vi "8Queen_quest2.vi"() -> ()   [LabVIEW 2012]
panel:
  out "Attempts":i32
  out "sec_past":dbl format="%#_4g"
  out "Solutions":i32
  in  "stop":bool
  in  "soln_dsp":i32=1
  out "board":bool[][](array[boolean])
  out "all_soln_out":i32[][](array[numeric])
  in  "Q_num":i32=9
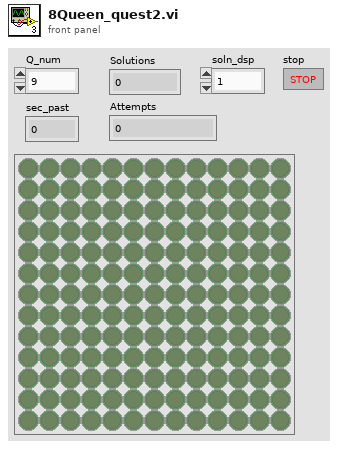
[diagram p1: front panel]
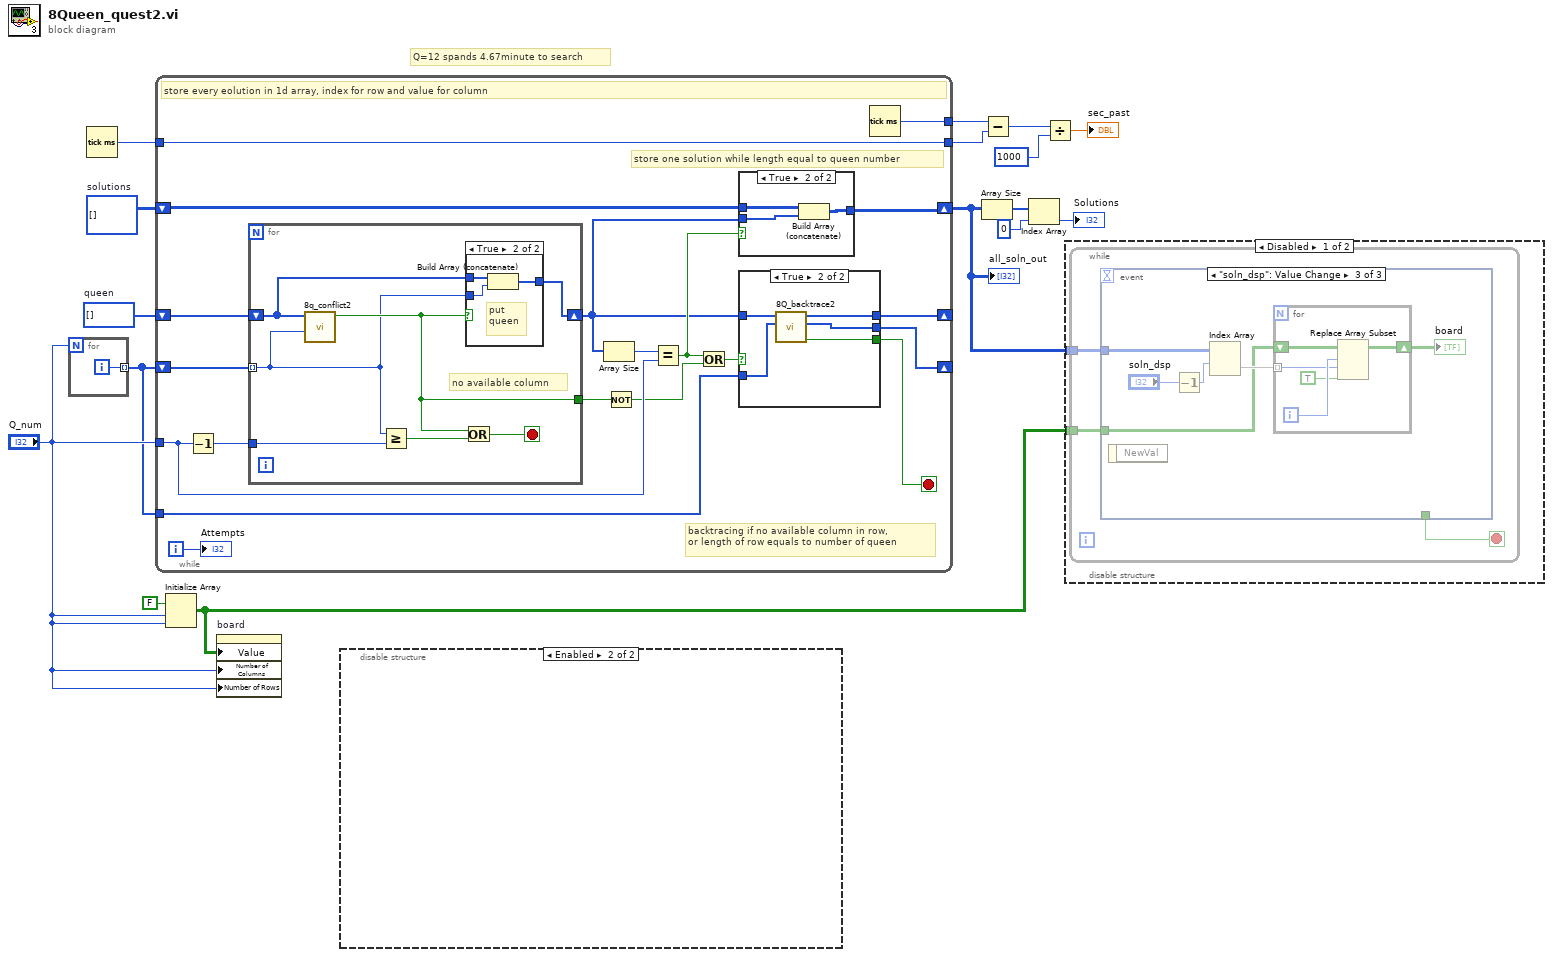
[diagram p0: block diagram]
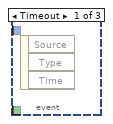
[diagram p2: hidden frame]
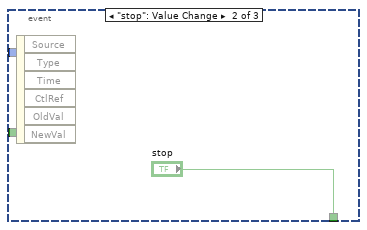
[diagram p3: hidden frame]
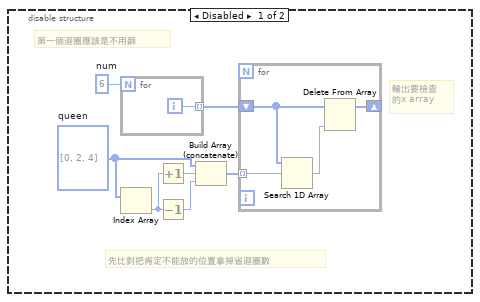
[diagram p5: hidden frame]
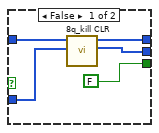
[diagram p8: hidden frame]
diagram:
  w15 = i32[] []  # queen
  w16 = i32[][] []  # solutions
  # "Q=12 spands 4.67minute to search"
  n1 = for {
    N: "Q_num" -> [_]
    tunnel: [w17] -> w1 mode=indexing
    i -> [w17]
  }
  n2 = Tick Count (ms)() -> (millisecond timer value=w4:u32)
  n3 = while {
    shift-right: [w33] -> _
    shift-left: w15 -> [w26]
    shift-right: [w27] -> _
    shift-left: w1 -> [w25]
    tunnel: "Q_num" -> [w31]
    shift-right: [w18] -> w14
    shift-left: w16 -> [w19]
    tunnel: [w30] -> w5
    tunnel: w4 -> [w29]
    tunnel: [w29] -> w3
    tunnel: w1 -> [w28]
    i -> [w22]
    stop <- w34 stop-if-true
    # "store one solution while length equal to queen number"
    # "backtracing if no available column in row,\nor length of row equals to number of queen"
    # "store every eolution in 1d array, index for row and value for column"
    n4 = Decrement(x=w31) -> (x-1=w32:i32)
    n5 = for {
      shift-right: [w41] -> w20
      shift-left: w26 -> [w42]
      tunnel: w32 -> [w47]
      tunnel: [w44] -> w23
      tunnel: w25 -> [w43] mode=indexing
      stop <- w45 stop-if-true
      # "no available column"
      n6 = call "8q_conflict2.vi"("nextX"=w43, "State"=w42) -> ("Available"=w44:bool)  [unwired: 9 in]
      n7 = Greater Or Equal?(x=w43, y=w47) -> (x >= y?=w46:bool)
      n8 = Or(x=w44, y=w46) -> (x .or. y?=w45:bool)
      n9 = case shown="True" w44 {
        tunnel: w43 -> [_ w51]
        tunnel: w42 -> [w48 w50]
        tunnel: [w48 w49] -> w41
        frame False {
        }
        frame True {
          # "put\nqueen"
          n10 = Build Array (concatenate)(w50, w51) -> (w49:i32[])
        }
      }
    }
    n11 = Array Size(array=w20) -> (size(s)=w36:i32)
    n12 = Not(x=w23) -> (.not. x?=w24:bool)
    n13 = Equal?(x=w36, y=w31) -> (x = y?=w21:bool)
    n14 = Or(x=w21, y=w24) -> (x .or. y?=w35:bool)
    n15 = case shown="True" w21 {
      tunnel: w20 -> [_ w40]
      tunnel: w19 -> [w37 w39]
      tunnel: [w37 w38] -> w18
      frame False {
      }
      frame True {
        n16 = Build Array (concatenate)(w39, w40) -> (w38:i32[][])
      }
    }
    n17 = case "backtracing" shown="True" w35 {
      tunnel: [w52 w59] -> w27
      tunnel: w20 -> [w54 w61]
      tunnel: [w53 w60] -> w33
      tunnel: [FALSE ("<0_stop") w58] -> w34
      tunnel: w28 -> [w55 w57]
      frame False {
        n18 = call "8q_kill CLR.vi"("nextX in"=w55, "queen in"=w54) -> ("nextX"=w52:i32[], "queen"=w53:i32[])  [unwired: 8 in]
      }
      frame True {
        n19 = call "8Q_backtrace2.vi"("all_x"=w57, "BT_bfr"=w61) -> ("<0_stop"=w58:bool, "next_start"=w59:i32[], "BT_result"=w60:i32[])  [unwired: 7 in]
      }
    }
    n20 = Tick Count (ms)() -> (millisecond timer value=w30:u32)
    "Attempts" <- w22
  }
  "all_soln_out" <- w14
  n21 = Initialize Array(FALSE, "Q_num", "Q_num") -> (w9:bool[][])
  n22 = property on="board" class="Arr (strict)"("Value"=w9, "Number of Columns"="Q_num", "Number of Rows"="Q_num") -> ()  [unwired: 2 in, 2 out]
  n23 = disable-structure shown="Enabled" {
    frame Disabled {
      w68 = 6  # num
      w65 = i32[] [0, 2, 4]  # queen
      # "第一個迴圈應該是不用篩"
      # "輸出要檢查\n的x array"
      # "先比對把肯定不能放的位置拿掉省迴圈數"
      n24 = for {
        N: w68 -> [_]
        tunnel: [w73] -> w67 mode=indexing
        i -> [w73]
      }
      n25 = Index Array(array=w65) -> (element=w63:i32)  [unwired: 1 in]
      n26 = Increment(x=w63) -> (x+1=w66:i32)
      n27 = Decrement(x=w63) -> (x-1=w64:i32)
      n28 = Build Array (concatenate)(w65, w66, w64) -> (w62:i32[])
      n29 = for {
        tunnel: w62 -> [w72] mode=indexing
        shift-right: [w69] -> _
        shift-left: w67 -> [w70]
        n30 = Search 1D Array(1D array=w70, element=w72) -> (index of element=w71:i32)  [unwired: 1 in]
        n31 = Delete From Array(array=w70, index=w71) -> (array with subset deleted=w69:i32[])  [unwired: 1 in, 1 out]
      }
    }
    frame Enabled {
    }
  }
  n32 = Array Size(array=w14) -> (size(s)=w13:i32[])
  n33 = Subtract(x=w5, y=w3) -> (x-y=w8:u32)
  n34 = Index Array(array=w13, index=0) -> (element=→"Solutions":i32)
  n35 = Divide(x=w8, y=u32 1000) -> (x/y=→"sec_past":dbl)
  n36 = disable-structure shown="Disabled" {
    disable-tunnel: w14 -> [w75 _]
    disable-tunnel: w9 -> [w74 _]
    frame Disabled {
      n37 = while {
        tunnel: w75 -> [w78]
        tunnel: w74 -> [w76]
        stop <- w77 stop-if-true
        n38 = event shown="[2] \"soln_dsp\": Value Change" {
          selector: _ -> [_ _ _]
          dyn-events: _ -> [_ _ _]
          timeout: _ -> [_ _ _]
          tunnel: w78 -> [_ _ w85]
          tunnel: [_ "stop" _] -> w77
          tunnel: w76 -> [_ _ w80]
          event Timeout {
            n39 = event-data() -> ()  [unwired: 1 in, 3 out]
          }
          event "stop": Value Change {
            n40 = event-data() -> ()  [unwired: 1 in, 6 out]
          }
          event "soln_dsp": Value Change {
            n41 = event-data() -> ()  [unwired: 1 in, 1 out]
            n42 = Decrement(x="soln_dsp") -> (x-1=w81:i32)
            n43 = Index Array(array=w85, index (row)=w81) -> (element=w84:i32[])  [unwired: 1 in]
            n44 = for {
              tunnel: w84 -> [w88] mode=indexing
              shift-right: [w87] -> w83
              shift-left: w80 -> [w90]
              i -> [w89]
              n45 = Replace Array Subset(array=w90, new element=TRUE, index (row)=w89, index (col)=w88) -> (w87:bool[][])
            }
            "board" <- w83
          }
        }
      }
    }
    frame Enabled {
    }
  }
